vi "Dashboard Main.vi"() -> ()   [LabVIEW 2012]
uses:
  <vilib>/Utility/config.llb/Read Key (String).vi
  <vilib>/Utility/config.llb/Read Key (I32).vi
  <vilib>/Utility/config.llb/Write Key (String).vi
  <vilib>/Utility/config.llb/Write Key (I32).vi
  <vilib>/Utility/config.llb/NI_LVConfig.lvlib
  Autonomous Selector/AutonomousSelector.lvlib
panel:
  out "Battery Value":dbl(slide) scale=0.0..14.0 scale format="%#_2e"
  out "Battery":sgl(graph)
  in  "Camera Settings":T1={"Frate Rate"=30, "Compression"=30, "Size"=1} {"Frate Rate" scale=1.0..30.0; "Size" items=["640x480", "320x240", "160x120"]}
  out "Mode":T2(ring)=enum."Auto Disabled"
  out "Camera IP":string
  out "JS1 Z":dbl(slide) scale=-1.0..1.0 scale format="%#_2e"
  out "JS2 Z":dbl(slide) scale=-1.0..1.0 scale format="%#_2e"
  out "Joystick 1":cluster{"X":dbl, "Y":dbl}[](graph)
  out "Joystick 2":cluster{"X":dbl, "Y":dbl}[](graph)
  out "JS Buttons 1":T3
  out "JS Buttons 2":T3
  out "MotorSlide4":dbl(slide) scale=-1.0..1.0 scale format="%#_2e"
  out "MotorSlide3":dbl(slide) scale=-1.0..1.0 scale format="%#_2e"
  out "MotorSlide2":dbl(slide) scale=-1.0..1.0 scale format="%#_2e"
  in  "MotorName3":string="Front Left"
  in  "MotorName4":string="Front Right"
  in  "MotorName1":string="Rear Left"
  in  "MotorName2":string="Rear Right"
  out "MotorChart4":dbl(graph)
  out "MotorChart3":dbl(graph)
  out "MotorChart2":dbl(graph)
  out "MotorSlide1":dbl(slide) scale=-1.0..1.0 scale format="%#_2e"
  out "MotorChart1":dbl(graph)
  out "Robot IP":string
  in  "Dashboard Tab":enum32{"Autonomous", "Test"}(tab)
  in  "Autonomous":u16(ring) items=["Do nothing", "Default autonomous", "My autonomous"]
  in  "Record":bool
  in  "Save":bool
  in  "Playback":bool
  in  "Slider":dbl(slide) scale=0.0..100.0 scale format="%#_3g"
  in  "On/Off":bool caption="Solenoid"
  in  "Test Name":u16(ring) items=["Select the test to run...", "Example Test", "-------------------------------", "List of tests is built in robot code.", "Replace with your own automated tests."]
  in  "Test Tree":string(tree)
  in  "Motor":cluster{"Value":dbl, "Enable":bool} {"Value" scale=-1.0..1.0 scale format="%#_3g"}
  out "Progress":T4 {"Test Progress" scale=0.0..100.0}
  in  "Rev/Fwd":cluster{"Forward":bool, "Reverse":bool}
  in  "Ring":u16(ring) items=["Auto", "Fixed indoor", "Fixed outdoor 1", "Fixed outdoor 2", "Fixed fluorescent 1", "Fixed fluorescent 2", "Hold current"]
  in  "Viewer":enum32{"Camera Image", "Variables"}(tab)
  out "Mbps":dbl format="%#.1g"
  in  "Enable":bool
  in  "DB Camera Config":bool
  out "Mbps":bool
  out "fps":dbl format="%#.1g"
  out "Image Error Message":string="Timeout in Camera Communications"
  out "Camera Image":T5(plugin-control)
  out "Tree":string(tree)
  # "Drive & Motors"
  # "Robot IP:"
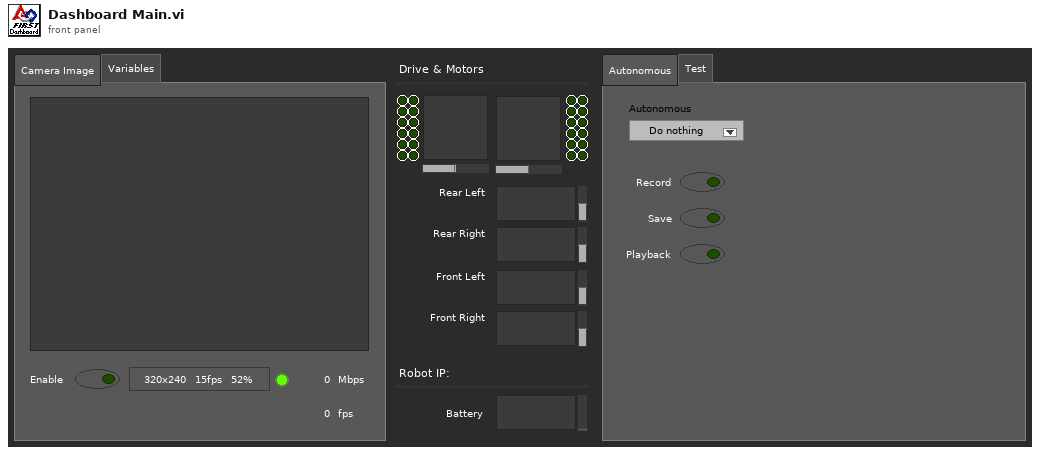
[diagram p1: front panel]
types:
  T1 = cluster{"Frate Rate":i32, "Compression":i32, "Size":u16}
  T2 = enum8{"Tele-Op Disabled", "Tele-Op Enabled", "Auto Disabled", "Auto Enabled", "Test Disabled", "Test Enabled", ""}
  T3 = cluster{bool, bool, bool, bool, bool, bool, bool, bool, bool, bool, bool, bool}
  T4 = cluster{"Test Progress":u8, "Test Progress Text":string}
  T5 = typedef "IMAQ Image.ctl" = refnum<image>
  T6 = typedef "Image Type" = u32
  T7 = typedef "LVRectTypeDef.ctl" = cluster{"Left":i16, "Top":i16, "Right":i16, "Bottom":i16}
  T8 = cluster{"Competition mode":bool, "Robot Link":bool, "Autonomous":bool, "Enabled":bool, "E-Stop":bool, "Simulated":bool, "TestMode":bool, "Docked Window":bool}
  T9 = cluster{"Boolean Array[0]":bool, "Boolean Array[1]":bool, "Boolean Array[2]":bool, "Boolean Array[3]":bool, "Boolean Array[4]":bool, "Boolean Array[5]":bool, "Boolean Array[6]":bool, "Boolean Array[7]":bool, "Boolean Array[8]":bool, "Boolean Array[9]":bool, "Boolean Array[10]":bool, "Boolean Array[11]":bool}
  T10 = typedef "NI_LVConfig.lvlib/Config Data RefNum.ctl" = refnum<k1>
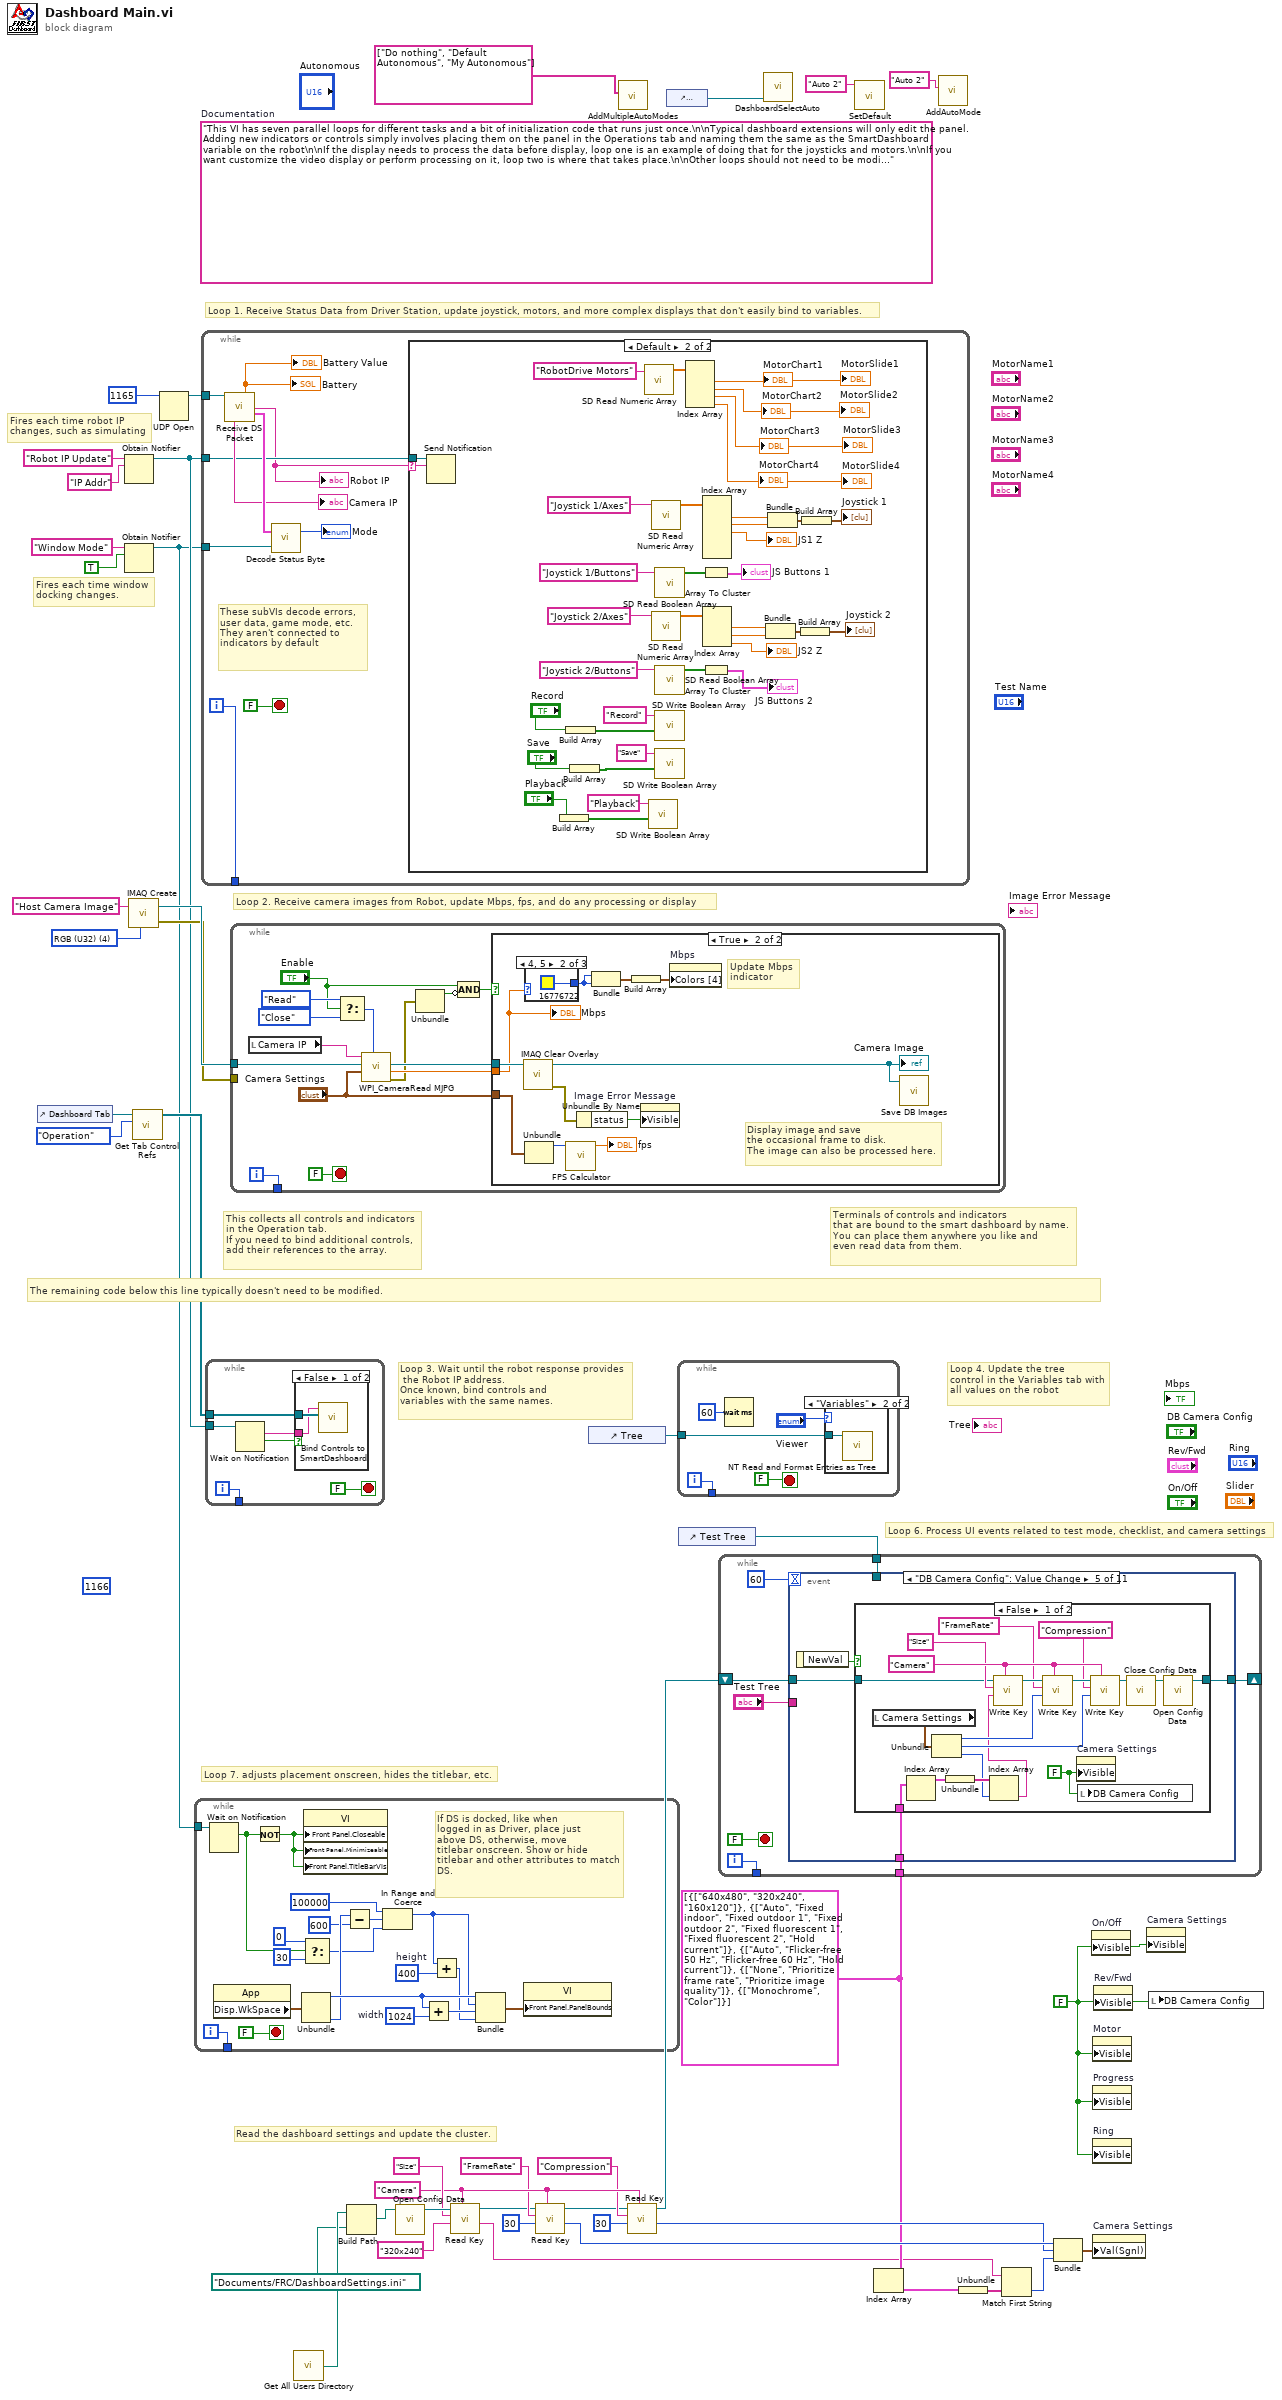
[diagram p0: block diagram]
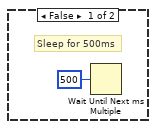
[diagram p3: hidden frame]
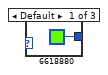
[diagram p4: hidden frame]
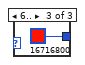
[diagram p5: hidden frame]
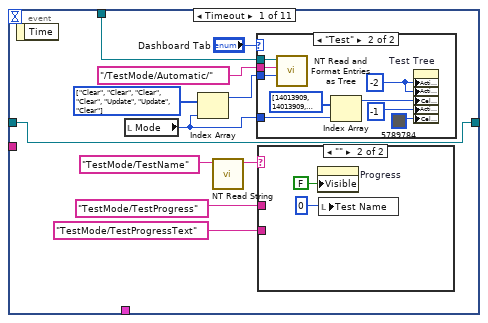
[diagram p6: hidden frame]
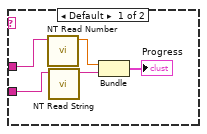
[diagram p8: hidden frame]
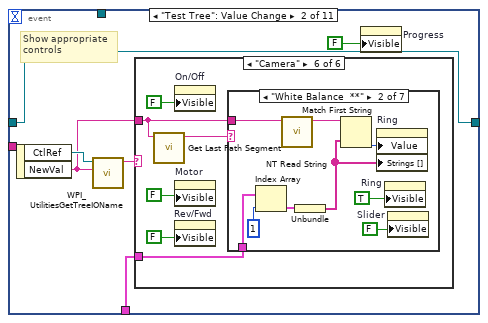
[diagram p9: hidden frame]
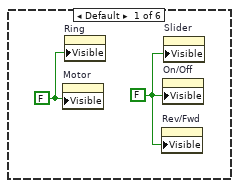
[diagram p10: hidden frame]
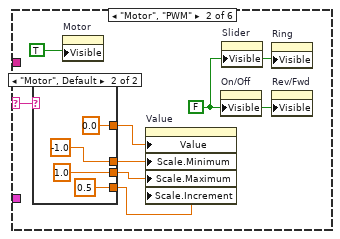
[diagram p11: hidden frame]
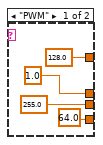
[diagram p12: hidden frame]
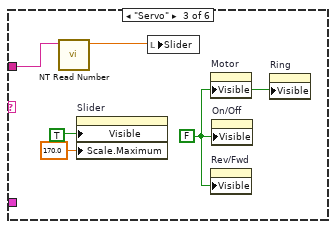
[diagram p13: hidden frame]
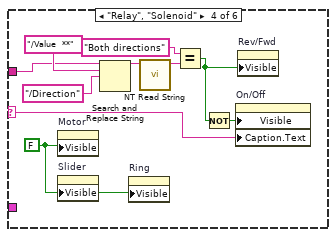
[diagram p14: hidden frame]
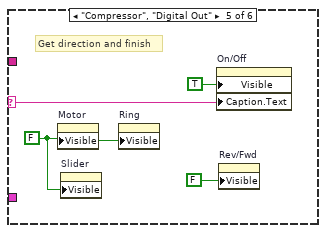
[diagram p15: hidden frame]
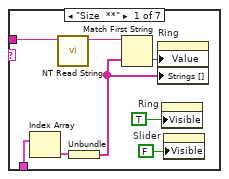
[diagram p16: hidden frame]
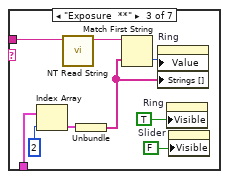
[diagram p17: hidden frame]
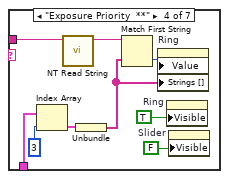
[diagram p18: hidden frame]
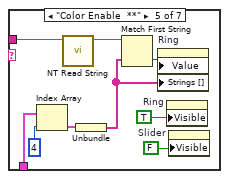
[diagram p19: hidden frame]
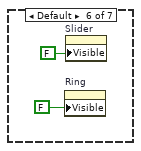
[diagram p20: hidden frame]
diagram:
  w23 = "Camera"
  w15 = cluster{string[]}[] [{["640x480", "320x240", "160x120"]}, {["Auto", "Fixed indoor", "Fixed outdoor 1", "Fixed outdoor 2", "Fixed fluorescent 1", "Fixed fluorescent 2", "Hold current"]}, {["Auto", "Flicker-free 50 Hz", "Flicker-free 60 Hz", "Hold current"]}, {["None", "Prioritize frame rate", "Prioritize image quality"]}, {["Monochrome", "Color"]}]
  w29 = FALSE ("Visible")
  (unwired) "This VI has seven parallel loops for different tasks and a bit of initialization code that runs just once.\n\nTypical dashboard extensions will only edit the panel. Adding new indicators or controls simply involves placing them on the panel in the Operations tab and naming them the same as the SmartDashboard variable on the robot\n\nIf the display needs to process the data before display, loop one is an example of doing that for the joysticks and motors.\n\nIf you want customize the video display or perform processing on it, loop two is where that takes place.\n\nOther loops should not need to be modified. They are pretty standard, and document the task they perform."  # Documentation
  (unwired) u16 1166 ("port")
  w42 = T6 4 items=["Grayscale (U8)", "Grayscale (I16)", "Grayscale (SGL)", "Complex (CSG)", "RGB (U32)", "HSL (U32)", "RGB (U64)"] ("Image Type")
  # "Fires each time robot IP\nchanges, such as simulating"
  # "Fires each time window\ndocking changes."
  # "This collects all controls and indicators\nin the Operation tab.\nIf you need to bind additional controls,\nadd their references to the array."
  # "The remaining code below this line typically doesn't need to be modified."
  # "Loop 6. Process UI events related to test mode, checklist, and camera settings"
  # "Read the dashboard settings and update the cluster."
  # "Terminals of controls and indicators\nthat are bound to the smart dashboard by name.\nYou can place them anywhere you like and\neven read data from them."
  # "Loop 4. Update the tree\ncontrol in the Variables tab with\nall values on the robot"
  # "Loop 3. Wait until the robot response provides\n the Robot IP address.\nOnce known, bind controls and\nvariables with the same names."
  # "Loop 7. adjusts placement onscreen, hides the titlebar, etc."
  # "Loop 1. Receive Status Data from Driver Station, update joystick, motors, and more complex displays that don't easily bind to variables."
  # "Loop 2. Receive camera images from Robot, update Mbps, fps, and do any processing or display"
  n1 = control-ref of="Dashboard Tab"() -> (w37:refnum<vi>)
  n2 = Obtain Notifier(name (unnamed)="Robot IP Update", notification data type="IP Addr" ("name (unnamed)")) -> (notifier out=w34:refnum<notifier>)  [unwired: 2 in, 2 out]
  n3 = Obtain Notifier(name (unnamed)="Window Mode", notification data type=TRUE) -> (notifier out=w30:refnum<notifier>)  [unwired: 2 in, 2 out]
  n4 = call "IMAQ Create"("Image Name"="Host Camera Image", "Image Type"=w42) -> ("New Image"=w40:T5, "error out"=w39:errorcluster)  [unwired: 2 in, 1 out]
  n5 = call <vilib>:"Get Tab Control Refs.vi"("Page Index"=enum32{"Operation", "Test"}."Operation" ("Dashboard Tab"), "TabControl in"=w37) -> ("ControlsOnPage"=w38:refnum<vi>[])  [unwired: 9 in]
  n6 = UDP Open(11:u16 1165 ("port")) -> (port=w43:refnum<k16>)  [unwired: 2 in, 4 out]
  n7 = while {
    tunnel: w30 -> [w63]
    tunnel: [w61] -> _
    i -> [w61]
    stop <- FALSE stop-if-true
    w53 = 1024  # width
    w56 = 400  # height
    # "If DS is docked, like when\nlogged in as Driver, place just\nabove DS, otherwise, move\ntitlebar onscreen. Show or hide\ntitlebar and other attributes to match\nDS."
    n8 = Wait on Notification(notifier=w63) -> (notification=w48:bool)  [unwired: 3 in, 3 out]
    n9 = property class="App"() -> ("Disp.WkSpace"=w59:T7)  [unwired: 2 in, 2 out]
    n10 = Not(x=w48) -> (.not. x?=w62:bool)
    n11 = Unbundle(w59) -> ("Left"=w57:i16, "Bottom"=w54:i16)  [unwired: 2 out]
    n12 = Select(t=0, s=w48, f=30) -> (s? t:f=w47:i32)
    n13 = property class="VI"("Front Panel.Closeable"=w62, "Front Panel.Minimizeable"=w62, "Front Panel.TitleBarVis"=w62) -> ()  [unwired: 2 in, 2 out]
    n14 = Subtract(x=w54, y=600) -> (x-y=w51:i32)
    n15 = In Range and Coerce(upper limit=100000, x=w51, lower limit=w47) -> (coerced(x)=w45:i32)  [unwired: 1 out]
    n16 = Add(x=w57, y=w53) -> (x+y=w58:i32)
    n17 = Add(x=w45, y=w56) -> (x+y=w55:i32)
    n18 = Bundle("Left"=w57, w45, w58, w55) -> (w60:cluster{"Left":i16, i32, i32, i32})  [unwired: 1 out]
    n19 = property class="VI"("Front Panel.PanelBounds"=w60) -> ()  [unwired: 2 in, 2 out]
  }
  n20 = while {
    tunnel: w43 -> [w72]
    tunnel: w34 -> [w66]
    tunnel: w30 -> [w70]
    tunnel: [w67] -> _
    i -> [w67]
    stop <- FALSE stop-if-true
    # "These subVIs decode errors, user data, game mode, etc.\nThey aren't connected to indicators by default"
    n21 = call "Receive DS Packet.vi"("Recv Socket"=w72) -> ("Battery"=→"Battery" →"Battery Value":sgl, "Robot IP Address"=w65:string, "Status"=w73:T8, "Camera IP Address"=→"Camera IP":string)  [unwired: 1 in, 10 out]
    "Robot IP" <- w65
    n22 = call "Decode Status Byte.vi"("Window Mode Notifier"=w70, "Status"=w73) -> ("Mode"=→"Mode":T2)  [unwired: 1 out]
    n23 = case shown="Default" w65 {
      selector: w65 -> [_ w84]
      tunnel: w66 -> [_ w85]
      frame "0.0.0.0" {
        # "Robot not responding, don't poll the variables"
      }
      frame Default {
        n24 = Send Notification(notification=w84, notifier=w85) -> ()  [unwired: 1 in, 2 out]
        n25 = Build Array("Playback") -> (w75:bool[])
        n26 = Build Array("Record") -> (w81:bool[])
        n27 = Build Array("Save") -> (w78:bool[])
        n28 = call <vilib>:"SD Read Numeric Array.vi"("Name"="RobotDrive Motors") -> ("Numeric Array"=w108:dbl[])  [unwired: 8 in, 2 out]
        n29 = call <vilib>:"SD Write Boolean Array.vi"("Boolean Array"=w75, "Name"="Playback") -> ()  [unwired: 8 in, 2 out]
        n30 = call <vilib>:"SD Read Numeric Array.vi"("Name"="Joystick 1/Axes") -> ("Numeric Array"=w101:dbl[])  [unwired: 8 in, 2 out]
        n31 = call <vilib>:"SD Read Numeric Array.vi"("Name"="Joystick 2/Axes") -> ("Numeric Array"=w95:dbl[])  [unwired: 8 in, 2 out]
        n32 = call <vilib>:"SD Read Boolean Array.vi"("Name"="Joystick 1/Buttons") -> ("Boolean Array"=w103:bool[])  [unwired: 8 in, 2 out]
        n33 = call <vilib>:"SD Read Boolean Array.vi"("Name"="Joystick 2/Buttons") -> ("Boolean Array"=w94:bool[])  [unwired: 8 in, 2 out]
        n34 = call <vilib>:"SD Write Boolean Array.vi"("Boolean Array"=w81, "Name"="Record") -> ()  [unwired: 8 in, 2 out]
        n35 = call <vilib>:"SD Write Boolean Array.vi"("Boolean Array"=w78, "Name"="Save") -> ()  [unwired: 8 in, 2 out]
        n36 = Index Array(array=w108) -> (element #1=→"MotorChart1" →"MotorSlide1":dbl, element #2=→"MotorSlide2" →"MotorChart2":dbl, element #3=→"MotorChart3" →"MotorSlide3":dbl, element #4=→"MotorChart4" →"MotorSlide4":dbl)  [unwired: 4 in]
        n37 = Array To Cluster(array=w103) -> (cluster=→"JS Buttons 1":T9)
        n38 = Array To Cluster(array=w94) -> (cluster=→"JS Buttons 2":T9)
        n39 = Index Array(array=w101) -> (element #1=w98:dbl, element #2=w99:dbl, element #3=→"JS1 Z":dbl)  [unwired: 6 in, 3 out]
        n40 = Index Array(array=w95) -> (element #1=w90:dbl, element #2=w89:dbl, element #3=→"JS2 Z":dbl)  [unwired: 3 in]
        n41 = Bundle("Numeric"=w90, "Numeric"=w89) -> (w91:cluster{"Numeric":dbl, "Numeric":dbl})  [unwired: 1 in]
        n42 = Bundle("Numeric"=w98, "Numeric"=w99) -> (w97:cluster{"Numeric":dbl, "Numeric":dbl})  [unwired: 1 in]
        n43 = Build Array(w91) -> (→"Joystick 2":cluster{"Numeric":dbl, "Numeric":dbl}[])
        n44 = Build Array(w97) -> (→"Joystick 1":cluster{"Numeric":dbl, "Numeric":dbl}[])
      }
    }
  }
  n45 = while {
    tunnel: w38 -> [w117]
    tunnel: w34 -> [w114]
    tunnel: [w112] -> _
    i -> [w112]
    stop <- FALSE stop-if-true
    n46 = Wait on Notification(notifier=w114) -> (notification=w113:string, timed out?=w115:bool)  [unwired: 3 in, 2 out]
    n47 = case shown="False" w115 {
      tunnel: w117 -> [w119 _]
      tunnel: w113 -> [w118 _]
      frame False {
        n48 = call <vilib>:"Bind Controls to SmartDashboard.vi"("Bound Control Refs"=w119, "Server IP Address"=w118) -> ()  [unwired: 10 in]
      }
      frame True {
      }
    }
  }
  n49 = while {
    tunnel: w40 -> [w129]
    tunnel: w39 -> [_]
    tunnel: [w132] -> _
    i -> [w132]
    stop <- FALSE stop-if-true
    n50 = local read "Camera IP"() -> (w131:string)
    n51 = Select(t=enum16{"Read", "Reopen", "Close"}."Read" ("Operation"), s="Enable", f=enum16{"Read", "Reopen", "Close"}."Close" ("Operation")) -> (s? t:f=w124:enum16{"Read", "Reopen", "Close"})
    n52 = call <vilib>:"WPI_CameraRead MJPG.vi"("Operation"=w124, "Camera Settings"="Camera Settings", "Image"=w129, "address"=w131) -> ("error out"=w123:errorcluster, "Bandwidth (kbps)"=w127:dbl, "Image Out"=w128:T5)  [unwired: 5 in]
    n53 = Unbundle(w123) -> ("status"=w121:bool)  [unwired: 2 out]
    n54 = Compound Arithmetic op=AND("Enable", invert w121) -> (w120:bool)
    n55 = case shown="True" w120 {
      tunnel: "Camera Settings" -> [_ w136]
      tunnel: w128 -> [_ w139]
      tunnel: w127 -> [_ w138]
      frame False {
        # "Sleep for 500ms"
        n56 = Wait Until Next ms Multiple(millisecond multiple=u32 500) -> ()  [unwired: 1 out]
      }
      frame True {
        # "Display image and save\nthe occasional frame to disk.\nThe image can also be processed here."
        # "Update Mbps\nindicator"
        n57 = call "IMAQ Clear Overlay"("Image"=w139) -> ("error out"=w144:errorcluster, "Image Out"=w143:T5)  [unwired: 2 in, 7 out]
        "Camera Image" <- w143
        n58 = case shown="4, 5" w138 {
          tunnel: [u32 6618880 ("Color Box") u32 16776722 ("Color Box") u32 16716800 ("Color Box")] -> w140
          frame Default {
          }
          frame 4, 5 {
          }
          frame 6.. {
          }
        }
        n59 = Unbundle(w136) -> ("Frate Rate"=w135:i32)  [unwired: 2 out]
        n60 = call "FPS Calculator.vi"("Average Count"=w135) -> ("fps"=→"fps":dbl)  [unwired: 10 in]
        n61 = Unbundle By Name(w144) -> ("status"=w145:bool)
        n62 = Bundle("Color Box"=w140, "Color Box"=w140) -> (w142:cluster{"Color Box":u32, "Color Box":u32})  [unwired: 1 out]
        n63 = Build Array(w142) -> (w141:cluster{"Color Box":u32, "Color Box":u32}[])
        n64 = property on="Image Error Message" class="Str"("Visible"=w145) -> ()  [unwired: 2 in, 2 out]
        n65 = property on="Mbps" class="Bool (strict)"("Colors [4]"=w141) -> ()  [unwired: 2 in, 2 out]
        n66 = call "Save DB Images.vi"("Image"=w143) -> ()  [unwired: 2 in, 1 out]
        "Mbps" <- w138
      }
    }
  }
  n67 = call "Get All Users Directory.vi"() -> ("All User Path"=w28:path)
  n68 = Build Path(base path=w28, name or relative path=path "Documents/FRC/DashboardSettings.ini") -> (appended path=w27:path)
  n69 = call <vilib>:"Open Config Data.vi"("configuration file path"=w27) -> ("refnum"=w26:T10)  [unwired: 8 in, 2 out]
  n70 = call-poly <vilib>:"Read Key.vi"("section"=w23, "default value"="320x240", "key"="Size", "refnum"=w26) -> ("value"=w13:string, "refnum out"=w10:T10)  [unwired: 2 in, 4 out]
  n71 = call-poly <vilib>:"Read Key.vi"("section"=w23, "default value"=30, "key"="FrameRate", "refnum"=w10) -> ("value"=w18:i32, "refnum out"=w9:T10)  [unwired: 1 in, 5 out]
  n72 = control-ref of="Tree"() -> (w6:refnum<vi>)
  n73 = call "AddMultipleAutoModes.vi"("Autonomous Modes"=string[] ["Do nothing", "Default Autonomous", "My Autonomous"]) -> ()  [unwired: 9 in, 1 out]
  n74 = call-poly <vilib>:"Read Key.vi"("section"=w23, "default value"=30, "key"="Compression", "refnum"=w9) -> ("value"=w17:i32, "refnum out"=w7:T10)  [unwired: 1 in, 5 out]
  n75 = control-ref of="Autonomous"() -> (w4:refnum<vi>)
  n76 = while {
    tunnel: [w150] -> _
    tunnel: w6 -> [w149]
    i -> [w150]
    stop <- FALSE stop-if-true
    n77 = Wait (ms)(milliseconds to wait=u32 60) -> ()  [unwired: 1 out]
    n78 = case shown="\"Variables\"" "Viewer" {
      tunnel: w149 -> [_ w154]
      frame Default {
      }
      frame "Variables" {
        n79 = call <vilib>:"NT Read and Format Entries as Tree.vi"("Tree Refnum"=w154) -> ()  [unwired: 9 in, 2 out]
      }
    }
  }
  n80 = control-ref of="Test Tree"() -> (w5:refnum<vi>)
  n81 = while {
    tunnel: w15 -> [w159]
    shift-right: [w158] -> _
    shift-left: w7 -> [w157]
    tunnel: [w156] -> _
    tunnel: w5 -> [w155]
    i -> [w156]
    stop <- FALSE stop-if-true
    n82 = event shown="[4] \"DB Camera Config\": Value Change" {
      selector: _ -> [_ _ _ _ _ _ _ _ _ _ _]
      dyn-events: _ -> [_ _ _ _ _ _ _ _ _ _ _]
      timeout: u32 60 ("milliseconds to wait") -> [_ _ _ _ _ _ _ _ _ _ _]
      tunnel: w155 -> [w169 _ _ _ _ _ _ _ _ _ _]
      tunnel: "Test Tree" -> [_ _ _ _ _ _ w339 w347 w349 w353 w361]
      tunnel: w159 -> [_ w191 _ _ w303 w333 _ _ _ _ _]
      tunnel: [w163 w190 _ w293 w302 w326 w338 w345 w348 w352 w360] -> w158
      tunnel: w157 -> [w163 w190 _ w293 w301 w326 w338 w345 w348 w352 w360]
      event Timeout {
        w168 = enum16{"Update", "Clear"}[] [enum."Clear", enum."Clear", enum."Clear", enum."Clear", enum."Update", enum."Update", enum."Clear"] items=["Update", "Clear"]
        n83 = event-data() -> ()  [unwired: 1 in, 1 out]
        n84 = local read "Mode"() -> (w166:T2)
        n85 = Index Array(array=w168, index=w166) -> (element=w167:enum16{"Update", "Clear"})
        n86 = call <vilib>:"NT Read String.vi"("Name"="TestMode/TestName") -> ("String"=w172:string)  [unwired: 9 in, 1 out]
        n87 = case shown="\"Test\"" "Dashboard Tab" {
          tunnel: w169 -> [_ w182]
          tunnel: "/TestMode/Automatic/" ("Name Pattern") -> [_ w181]
          tunnel: w167 -> [_ w180]
          tunnel: w166 -> [_ w178]
          frame "Autonomous", Default {
          }
          frame "Test" {
            w177 = -2 ("Active Item:Row Number")
            n88 = call <vilib>:"NT Read and Format Entries as Tree.vi"("Operation"=w180, "Name Pattern"=w181, "Tree Refnum"=w182) -> ()  [unwired: 7 in, 2 out]
            n89 = Index Array(array=u32[] [14013909, 14013909, 14013909, 14013909, 14013909, 16777215, 14013909], index=w178) -> (element=w176:u32)
            n90 = property on="Test Tree" class="Tree (strict)"("Active Item Row Number"=w177, "ActiveColNum"=w177, "CellBG"=w176, "Active Item Row Number"=-1 ("Active Item:Row Number"), "CellBG"=u32 5789784 ("Color Box")) -> ()  [unwired: 2 in, 2 out]
          }
        }
        n91 = case shown="\"\"" w172 {
          tunnel: "TestMode/TestProgress" ("Name") -> [w184 _]
          tunnel: "TestMode/TestProgressText" ("Name") -> [w183 _]
          frame Default {
            n92 = call <vilib>:"NT Read Number.vi"("Name"=w184) -> ("Numeric"=w185:dbl)  [unwired: 9 in, 1 out]
            n93 = call <vilib>:"NT Read String.vi"("Name"=w183) -> ("String"=w186:string)  [unwired: 9 in, 1 out]
            n94 = Bundle("Numeric"=w185, "String"=w186) -> (→"Progress":cluster{"Numeric":dbl, "String":string})  [unwired: 1 in]
          }
          frame "" {
            n95 = property on="Progress" class="Clust (strict)"("Visible"=FALSE) -> ()  [unwired: 2 in, 2 out]
            n96 = local write "Test Name"(u16 0) -> ()
          }
        }
      }
      event "Test Tree": Value Change {
        # "Show appropriate\ncontrols"
        n97 = event-data() -> ("CtlRef"=w194:refnum<vi>, "NewVal"=w192:string)  [unwired: 1 in]
        n98 = call <vilib>:"WPI_UtilitiesGetTreeIOName.vi"("NewVal"=w192, "TreeControl in"=w194) -> ("I/O Name"=w195:string)  [unwired: 9 in]
        n99 = case shown="\"Camera\"" w195 {
          selector: w195 -> [_ w202 _ w220 w229 _]
          tunnel: w192 -> [_ _ w217 w219 _ w236]
          tunnel: w191 -> [_ _ _ _ _ w235]
          frame Default {
            w197 = FALSE ("Visible")
            w196 = FALSE ("Visible")
            n100 = property on="Motor" class="Clust (strict)"("Visible"=w196) -> ()  [unwired: 2 in, 2 out]
            n101 = property on="Ring" class="Ring (strict)"("Visible"=w196) -> ()  [unwired: 2 in, 2 out]
            n102 = property on="Rev/Fwd" class="Clust (strict)"("Visible"=w197) -> ()  [unwired: 2 in, 2 out]
            n103 = property on="On/Off" class="Bool (strict)"("Visible"=w197) -> ()  [unwired: 2 in, 2 out]
            n104 = property on="Slider" class="Slide (strict)"("Visible"=w197) -> ()  [unwired: 2 in, 2 out]
          }
          frame "Motor", "PWM" {
            w203 = FALSE ("Visible")
            n105 = case shown="\"Motor\", Default" w202 {
              tunnel: [1.0 ("Value") -1.0 ("Value")] -> w201
              tunnel: [255.0 ("Value") 1.0 ("Value")] -> w200
              tunnel: [128.0 ("Value") 0.0 ("Value")] -> w199
              tunnel: [64.0 ("Value") 0.5 ("Value")] -> w198
              frame "PWM" {
              }
              frame "Motor", Default {
              }
            }
            n106 = property on="Motor" class="Clust (strict)"("Visible"=TRUE) -> ()  [unwired: 2 in, 2 out]
            n107 = property on="Value" class="Slide (strict)"("Value"=w199, "Scale.Minimum"=w201, "Scale.Maximum"=w200, "Scale.Increment"=w198) -> ()  [unwired: 2 in, 2 out]
            n108 = property on="On/Off" class="Bool (strict)"("Visible"=w203) -> ()  [unwired: 2 in, 2 out]
            n109 = property on="Slider" class="Slide (strict)"("Visible"=w203) -> ()  [unwired: 2 in, 2 out]
            n110 = property on="Ring" class="Ring (strict)"("Visible"=w203) -> ()  [unwired: 2 in, 2 out]
            n111 = property on="Rev/Fwd" class="Clust (strict)"("Visible"=w203) -> ()  [unwired: 2 in, 2 out]
          }
          frame "Servo" {
            w215 = FALSE ("Visible")
            n112 = call <vilib>:"NT Read Number.vi"("Name"=w217) -> ("Numeric"=w216:dbl)  [unwired: 9 in, 1 out]
            n113 = property on="Slider" class="Slide (strict)"("Visible"=TRUE, "Scale.Maximum"=170.0 ("Scale.Range:Maximum")) -> ()  [unwired: 2 in, 2 out]
            n114 = local write "Slider"(w216) -> ()
            n115 = property on="Motor" class="Clust (strict)"("Visible"=w215) -> ()  [unwired: 2 in, 2 out]
            n116 = property on="Rev/Fwd" class="Clust (strict)"("Visible"=w215) -> ()  [unwired: 2 in, 2 out]
            n117 = property on="On/Off" class="Bool (strict)"("Visible"=w215) -> ()  [unwired: 2 in, 2 out]
            n118 = property on="Ring" class="Ring (strict)"("Visible"=w215) -> ()  [unwired: 2 in, 2 out]
          }
          frame "Relay", "Solenoid" {
            w218 = FALSE ("Visible")
            n119 = property on="Motor" class="Clust (strict)"("Visible"=w218) -> ()  [unwired: 2 in, 2 out]
            n120 = property on="Slider" class="Slide (strict)"("Visible"=w218) -> ()  [unwired: 2 in, 2 out]
            n121 = Search and Replace String(input string=w219, search string="/Value  **", replace string="/Direction") -> (result string=w225:string)  [unwired: 5 in, 3 out]
            n122 = property on="Ring" class="Ring (strict)"("Visible"=w218) -> ()  [unwired: 2 in, 2 out]
            n123 = call <vilib>:"NT Read String.vi"("Name"=w225) -> ("String"=w223:string)  [unwired: 9 in, 1 out]
            n124 = Equal?(x="Both directions", y=w223) -> (x = y?=w221:bool)
            n125 = Not(x=w221) -> (.not. x?=w222:bool)
            n126 = property on="On/Off" class="Bool (strict)"("Visible"=w222, "Caption.Text"=w220) -> ()  [unwired: 2 in, 2 out]
            n127 = property on="Rev/Fwd" class="Clust (strict)"("Visible"=w221) -> ()  [unwired: 2 in, 2 out]
          }
          frame "Compressor", "Digital Out" {
            w228 = FALSE ("Visible")
            # "Get direction and finish"
            n128 = property on="Motor" class="Clust (strict)"("Visible"=w228) -> ()  [unwired: 2 in, 2 out]
            n129 = property on="Slider" class="Slide (strict)"("Visible"=w228) -> ()  [unwired: 2 in, 2 out]
            n130 = property on="Ring" class="Ring (strict)"("Visible"=w228) -> ()  [unwired: 2 in, 2 out]
            n131 = property on="On/Off" class="Bool (strict)"("Visible"=TRUE, "Caption.Text"=w229) -> ()  [unwired: 2 in, 2 out]
            n132 = property on="Rev/Fwd" class="Clust (strict)"("Visible"=FALSE) -> ()  [unwired: 2 in, 2 out]
          }
          frame "Camera" {
            n133 = call <vilib>:"Get Last Path Segment.vi"("String in"=w236) -> ("String out"=w237:string)  [unwired: 10 in]
            n134 = property on="On/Off" class="Bool (strict)"("Visible"=FALSE) -> ()  [unwired: 2 in, 2 out]
            n135 = property on="Motor" class="Clust (strict)"("Visible"=FALSE) -> ()  [unwired: 2 in, 2 out]
            n136 = property on="Rev/Fwd" class="Clust (strict)"("Visible"=FALSE) -> ()  [unwired: 2 in, 2 out]
            n137 = case shown="\"White Balance  **\"" w237 {
              tunnel: w236 -> [w243 w252 w261 w270 w279 _ w285]
              tunnel: w235 -> [w241 w249 w258 w267 w276 _ _]
              frame "Size  **" {
                n138 = Index Array(array=w241) -> (element=w240:cluster{string[]})  [unwired: 1 in]
                n139 = call <vilib>:"NT Read String.vi"("Name"=w243) -> ("String"=w242:string)  [unwired: 9 in, 1 out]
                n140 = Unbundle(w240) -> (w238:string[])
                n141 = Match First String(2:w238, 3:w242) -> (0:w239:i32)  [unwired: 1 out]
                n142 = property on="Ring" class="Ring (strict)"("Value"=w239, "Strings []"=w238) -> ()  [unwired: 2 in, 2 out]
                n143 = property on="Ring" class="Ring (strict)"("Visible"=TRUE) -> ()  [unwired: 2 in, 2 out]
                n144 = property on="Slider" class="Slide (strict)"("Visible"=FALSE) -> ()  [unwired: 2 in, 2 out]
              }
              frame "White Balance  **" {
                n145 = Index Array(array=w249, index=1) -> (element=w250:cluster{string[]})
                n146 = call <vilib>:"NT Read String.vi"("Name"=w252) -> ("String"=w251:string)  [unwired: 9 in, 1 out]
                n147 = Unbundle(w250) -> (w247:string[])
                n148 = Match First String(2:w247, 3:w251) -> (0:w246:i32)  [unwired: 1 out]
                n149 = property on="Ring" class="Ring (strict)"("Value"=w246, "Strings []"=w247) -> ()  [unwired: 2 in, 2 out]
                n150 = property on="Ring" class="Ring (strict)"("Visible"=TRUE) -> ()  [unwired: 2 in, 2 out]
                n151 = property on="Slider" class="Slide (strict)"("Visible"=FALSE) -> ()  [unwired: 2 in, 2 out]
              }
              frame "Exposure  **" {
                n152 = Index Array(array=w258, index=2) -> (element=w259:cluster{string[]})
                n153 = call <vilib>:"NT Read String.vi"("Name"=w261) -> ("String"=w260:string)  [unwired: 9 in, 1 out]
                n154 = Unbundle(w259) -> (w255:string[])
                n155 = Match First String(2:w255, 3:w260) -> (0:w256:i32)  [unwired: 1 out]
                n156 = property on="Ring" class="Ring (strict)"("Value"=w256, "Strings []"=w255) -> ()  [unwired: 2 in, 2 out]
                n157 = property on="Ring" class="Ring (strict)"("Visible"=TRUE) -> ()  [unwired: 2 in, 2 out]
                n158 = property on="Slider" class="Slide (strict)"("Visible"=FALSE) -> ()  [unwired: 2 in, 2 out]
              }
              frame "Exposure Priority  **" {
                n159 = Index Array(array=w267, index=3) -> (element=w268:cluster{string[]})
                n160 = call <vilib>:"NT Read String.vi"("Name"=w270) -> ("String"=w269:string)  [unwired: 9 in, 1 out]
                n161 = Unbundle(w268) -> (w264:string[])
                n162 = Match First String(2:w264, 3:w269) -> (0:w265:i32)  [unwired: 1 out]
                n163 = property on="Ring" class="Ring (strict)"("Value"=w265, "Strings []"=w264) -> ()  [unwired: 2 in, 2 out]
                n164 = property on="Ring" class="Ring (strict)"("Visible"=TRUE) -> ()  [unwired: 2 in, 2 out]
                n165 = property on="Slider" class="Slide (strict)"("Visible"=FALSE) -> ()  [unwired: 2 in, 2 out]
              }
              frame "Color Enable  **" {
                n166 = Index Array(array=w276, index=4) -> (element=w277:cluster{string[]})
                n167 = call <vilib>:"NT Read String.vi"("Name"=w279) -> ("String"=w278:string)  [unwired: 9 in, 1 out]
                n168 = Unbundle(w277) -> (w273:string[])
                n169 = Match First String(2:w273, 3:w278) -> (0:w274:i32)  [unwired: 1 out]
                n170 = property on="Ring" class="Ring (strict)"("Value"=w274, "Strings []"=w273) -> ()  [unwired: 2 in, 2 out]
                n171 = property on="Ring" class="Ring (strict)"("Visible"=TRUE) -> ()  [unwired: 2 in, 2 out]
                n172 = property on="Slider" class="Slide (strict)"("Visible"=FALSE) -> ()  [unwired: 2 in, 2 out]
              }
              frame Default {
                n173 = property on="Ring" class="Ring (strict)"("Visible"=FALSE) -> ()  [unwired: 2 in, 2 out]
                n174 = property on="Slider" class="Slide (strict)"("Visible"=FALSE) -> ()  [unwired: 2 in, 2 out]
              }
              frame "Brightness  **", "Color Level  **", "Compression  **", "FPS  **", "Sharpness  **" {
                n175 = call <vilib>:"NT Read Number.vi"("Name"=w285) -> ("Numeric"=w284:dbl)  [unwired: 9 in, 1 out]
                n176 = local write "Slider"(w284) -> ()
                n177 = property on="Slider" class="Slide (strict)"("Visible"=TRUE, "Scale.Maximum"=100.0 ("Scale.Range:Maximum")) -> ()  [unwired: 2 in, 2 out]
                n178 = property on="Ring" class="Ring (strict)"("Visible"=FALSE) -> ()  [unwired: 2 in, 2 out]
              }
            }
          }
        }
        n179 = property on="Progress" class="Clust (strict)"("Visible"=FALSE) -> ()  [unwired: 2 in, 2 out]
      }
      event "Test Name": Mouse Enter {
        # "Populate the ring with the list of tests"
        n180 = event-data() -> ()  [unwired: 1 in, 1 out]
        n181 = call <vilib>:"NT Read String Array.vi"("Name"="TestMode/TestList") -> ("String Array"=w292:string[])  [unwired: 9 in, 1 out]
        n182 = Build Array (concatenate)("Select the test to run...", w292) -> (w291:string[])
        n183 = property on="Test Name" class="Ring (strict)"("Strings []"=w291) -> ()  [unwired: 2 in, 2 out]
      }
      event "Test Name": Value Change {
        w294 = FALSE ("Visible")
        # "Tell the robot the test name to run"
        n184 = event-data() -> ("NewVal"=w298:u16)  [unwired: 1 in]
        n185 = property on="Test Name" class="Ring (strict)"() -> ("Strings []"=w299:string[])  [unwired: 2 in, 2 out]
        n186 = local write "Progress"(T4 {"Test Progress"=0, "Test Progress Text"=""} ("Progress")) -> ()
        n187 = Index Array(array=w299, index=w298) -> (element=w297:string)
        n188 = call <vilib>:"NT Write String.vi"("String"=w297, "Name"="TestMode/TestName") -> ()  [unwired: 9 in, 1 out]
        n189 = property on="Progress" class="Clust (strict)"("Visible"=TRUE) -> ()  [unwired: 2 in, 2 out]
        n190 = property on="Motor" class="Clust (strict)"("Visible"=w294) -> ()  [unwired: 2 in, 2 out]
        n191 = property on="Slider" class="Slide (strict)"("Visible"=w294) -> ()  [unwired: 2 in, 2 out]
        n192 = property on="On/Off" class="Bool (strict)"("Visible"=w294) -> ()  [unwired: 2 in, 2 out]
        n193 = property on="Rev/Fwd" class="Clust (strict)"("Visible"=w294) -> ()  [unwired: 2 in, 2 out]
        n194 = property on="Ring" class="Ring (strict)"("Visible"=w294) -> ()  [unwired: 2 in, 2 out]
      }
      event "DB Camera Config": Value Change {
        n195 = event-data() -> ("NewVal"=w304:bool)  [unwired: 1 in]
        n196 = case shown="False" w304 {
          tunnel: w303 -> [w313 _]
          tunnel: [w306 w324] -> w302
          tunnel: w301 -> [w305 w324]
          frame False {
            w320 = "Camera"
            w323 = FALSE ("Visible")
            n197 = local read "Camera Settings"() -> (w312:T1)
            n198 = Index Array(array=w313) -> (element=w316:cluster{string[]})  [unwired: 1 in]
            n199 = Unbundle(w312) -> ("Frate Rate"=w311:i32, "Compression"=w310:i32, "Size"=w314:u16)
            n200 = Unbundle(w316) -> (w315:string[])
            n201 = Index Array(array=w315, index=w314) -> (element=w309:string)
            n202 = call-poly <vilib>:"Write Key.vi"("section"=w320, "value"=w309, "key"="Size", "refnum"=w305) -> ("refnum out"=w322:T10)  [unwired: 2 in, 5 out]
            n203 = call-poly <vilib>:"Write Key.vi"("section"=w320, "value"=w311, "key"="FrameRate", "refnum"=w322) -> ("refnum out"=w321:T10)  [unwired: 1 in, 6 out]
            n204 = property on="Camera Settings" class="Clust (strict)"("Visible"=w323) -> ()  [unwired: 2 in, 2 out]
            n205 = local write "DB Camera Config"(w323) -> ()
            n206 = call-poly <vilib>:"Write Key.vi"("section"=w320, "value"=w310, "key"="Compression", "refnum"=w321) -> ("refnum out"=w307:T10)  [unwired: 1 in, 6 out]
            n207 = call <vilib>:"Close Config Data.vi"("refnum"=w307) -> ("file path"=w308:path)  [unwired: 2 in, 8 out]
            n208 = call <vilib>:"Open Config Data.vi"("configuration file path"=w308) -> ("refnum"=w306:T10)  [unwired: 8 in, 2 out]
          }
          frame True {
            n209 = property on="Camera Settings" class="Clust (strict)"("Visible"=TRUE) -> ()  [unwired: 2 in, 2 out]
          }
        }
      }
      event "Camera Settings": Value Change {
        n210 = event-data() -> ("NewVal"=w337:T1)  [unwired: 1 in]
        n211 = Index Array(array=w333) -> (element=w332:cluster{string[]})  [unwired: 1 in]
        n212 = Unbundle(w337) -> ("Frate Rate"=w328:i32, "Compression"=w327:i32, "Size"=w330:u16)
        n213 = Unbundle(w332) -> (w331:string[])
        n214 = Index Array(array=w331, index=w330) -> (element=w329:string)
        n215 = Format Into String(format string="%s   %dfps   %d%%", w329, w328, w327) -> (resulting string=w334:string)  [unwired: 2 in, 1 out]
        n216 = Build Array(w334) -> (w335:string[])
        n217 = property on="DB Camera Config" class="Bool (strict)"("Strings [4]"=w335) -> ()  [unwired: 2 in, 2 out]
      }
      event "Motor.Enable": Value Change {
        n218 = event-data() -> ("NewVal"=w343:bool)  [unwired: 1 in]
        n219 = Unbundle("Motor") -> ("Value"=w342:dbl)  [unwired: 1 out]
        n220 = Select(t=w342, s=w343, f=0.0) -> (s? t:f=w340:dbl)
        n221 = call <vilib>:"NT Write Number.vi"("Numeric"=w340, "Name"=w339) -> ()  [unwired: 9 in, 1 out]
      }
      event "Slider": Value Change {
        n222 = event-data() -> ("NewVal"=w346:dbl)  [unwired: 1 in]
        n223 = call <vilib>:"NT Write Number.vi"("Numeric"=w346, "Name"=w347) -> ()  [unwired: 9 in, 1 out]
      }
      event "On/Off": Value Change {
        n224 = event-data() -> ("NewVal"=w351:bool)  [unwired: 1 in]
        n225 = Boolean To (0,1)(Boolean=w351) -> (0, 1=w350:i16)
        n226 = call <vilib>:"NT Write Number.vi"("Numeric"=w350, "Name"=w349) -> ()  [unwired: 9 in, 1 out]
      }
      event "Rev/Fwd": Value Change {
        n227 = event-data() -> ("NewVal.Forward"=w359:bool, "NewVal.Reverse"=w358:bool)  [unwired: 1 in]
        n228 = Boolean To (0,1)(Boolean=w359) -> (0, 1=w355:i16)
        n229 = Boolean To (0,1)(Boolean=w358) -> (0, 1=w357:i16)
        n230 = Negate(x=w357) -> (-x=w356:i16)
        n231 = Add(x=w355, y=w356) -> (x+y=w354:i16)
        n232 = call <vilib>:"NT Write Number.vi"("Numeric"=w354, "Name"=w353) -> ()  [unwired: 9 in, 1 out]
      }
      event "Ring": Value Change {
        n233 = event-data() -> ("NewVal"=w363:u16)  [unwired: 1 in]
        n234 = property on="Ring" class="Ring (strict)"() -> ("Strings []"=w364:string[])  [unwired: 2 in, 2 out]
        n235 = Index Array(array=w364, index=w363) -> (element=w362:string)
        n236 = call <vilib>:"NT Write String.vi"("String"=w362, "Name"=w361) -> ()  [unwired: 9 in, 1 out]
      }
    }
  }
  n237 = call "DashboardSelectAuto.vi"("Autonomous Mode Ring"=w4) -> ()  [unwired: 10 in]
  n238 = call "SetDefault.vi"("Table Prefix"="Auto 2") -> ()  [unwired: 9 in, 1 out]
  n239 = Index Array(array=w15) -> (element=w16:cluster{string[]})  [unwired: 1 in]
  n240 = call "AddAutoMode.vi"("Autonomous Mode"="Auto 2" ("Table Prefix")) -> ()  [unwired: 9 in, 1 out]
  n241 = Unbundle(w16) -> (w14:string[])
  n242 = Match First String(2:w14, 3:w13) -> (0:w12:i32)  [unwired: 1 out]
  n243 = Bundle("value"=w18, "value"=w17, "index"=w12) -> (w8:cluster{"value":i32, "value":i32, "index":i32})  [unwired: 1 out]
  n244 = property on="On/Off" class="Bool (strict)"("Visible"=w29) -> ()  [unwired: 2 in, 2 out]
  n245 = property on="Motor" class="Clust (strict)"("Visible"=w29) -> ()  [unwired: 2 in, 2 out]
  n246 = property on="Progress" class="Clust (strict)"("Visible"=w29) -> ()  [unwired: 2 in, 2 out]
  n247 = property on="Ring" class="Ring (strict)"("Visible"=w29) -> ()  [unwired: 2 in, 2 out]
  n248 = property on="Camera Settings" class="Clust (strict)"("Val(Sgnl)"=w8) -> ()  [unwired: 2 in, 2 out]
  n249 = property on="Rev/Fwd" class="Clust (strict)"("Visible"=w29) -> ()  [unwired: 2 in, 2 out]
  n250 = property on="Camera Settings" class="Clust (strict)"("Visible"=w29) -> ()  [unwired: 2 in, 2 out]
  n251 = local write "DB Camera Config"(w29) -> ()
